vi "MeasurementEnded Event Callback.vi"(4 "User Parameter":T1, 5 "Event Data":cluster{"sender":refnum<k24>, "e":refnum<k24>}, 6 "Control Ref":refnum<k24>, 7 "Event Common Data":T2) -> ()   [LabVIEW 2025]
uses:
  E:/PSCode/PalmSens_SDK/labview/PalmSens/Libraries/PalmSens.Core.Simplified.LabVIEW.dll
  Libraries/PalmSens.Core.Simplified.LabVIEW.dll
  MeasurementEventArgs.ctl
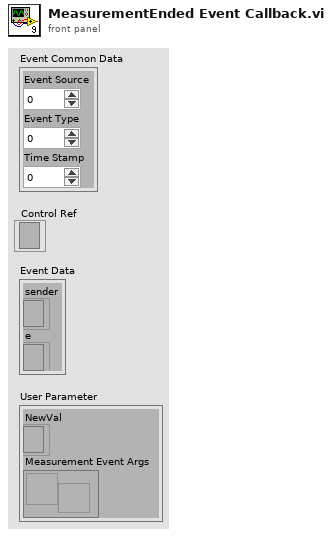
[diagram p1: front panel]
types:
  T1 = cluster{"NewVal":refnum<k24>, "Measurement Event Args":refnum<user-event>}
  T2 = cluster{"Event Source":i32, "Event Type":u32, "Time Stamp":u32}
  T3 = typedef "MeasurementEventArgs.ctl" = cluster{"Active Measurement":refnum<k24>, "Dispose":bool}
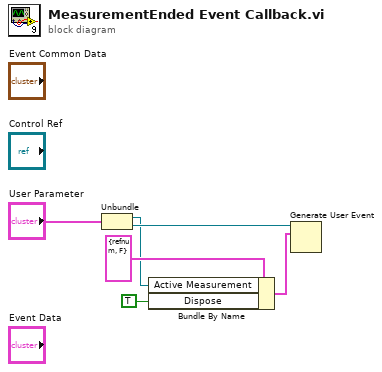
[diagram p0: block diagram]
diagram:
  n1 = Unbundle("User Parameter") -> ("NewVal"=w3:refnum<k24>, "Measurement Event Args"=w5:refnum<user-event>)
  n2 = Bundle By Name(cluster=T3 {"Active Measurement"=refnum, "Dispose"=FALSE} ("Measurement Ended Event Args"), "Active Measurement"=w3, "Dispose"=TRUE) -> (w2:T3)
  n3 = Generate User Event(user event=w5, event data cluster=w2) -> ()  [unwired: 2 in, 2 out]
